vi "Init_UI_Buttons.vi"(0 "VISAResourceName in":refnum<vi>, 1 "Enum Refnum":refnum<vi>, 2 "Bool Refnum 2":refnum<vi>, 3 "Bool Refnum":refnum<vi>, 5 "Str Refnum":refnum<vi>, 7 "DigNum Refnum":refnum<vi>, 9 "DigNum Refnum 2":refnum<vi>, 11 "error in (no error)":errorcluster, 12 "DigNum Refnum 3":refnum<vi>, 13 "Ring Refnum":refnum<vi>) -> (15 "error out":errorcluster)   [LabVIEW 2023, in "TranslationStage Library.lvlib" / "TranslationStage_UI.lvlib" / "TranslationStageUI.lvclass"]
uses:
  TranslationStageUI.lvclass
  TranslationStageUI.lvclass/TranslationStageUI.ctl
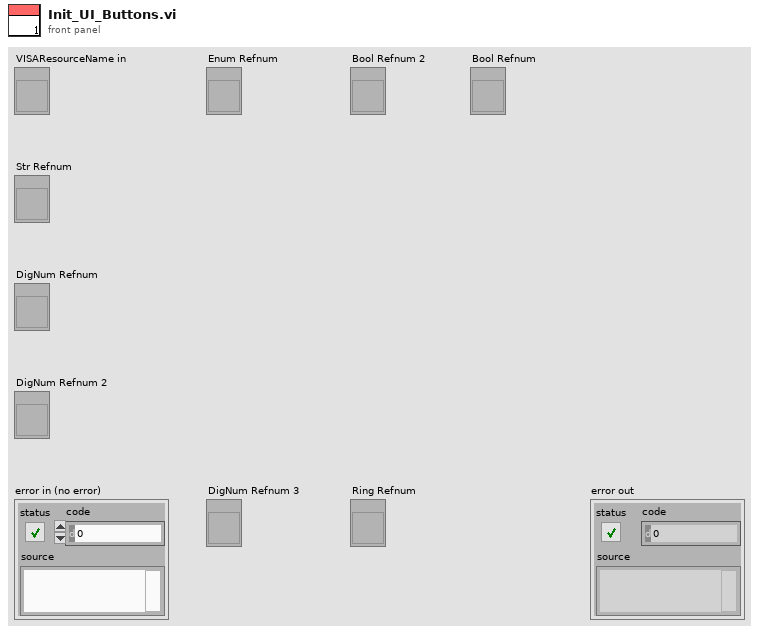
[diagram p1: front panel]
types:
  T1 = enum8{"Enabled", "Disabled", "Disabled and Grayed Out"}
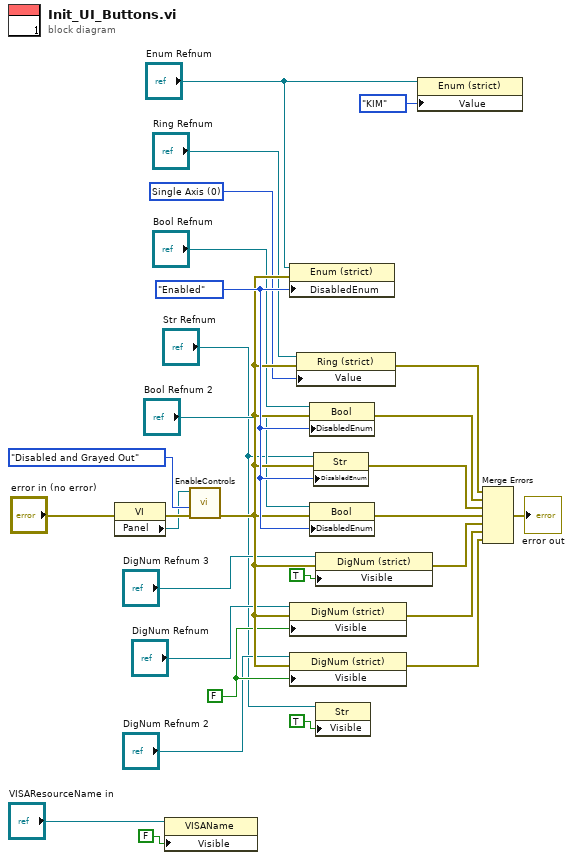
[diagram p0: block diagram]
diagram:
  w16 = 0 items=["Single Axis", "Raster"] ("Scan Mode")
  w15 = FALSE ("Visible")
  w26 = T1."Enabled" ("Disabled")
  n1 = property class="VI"(error in="error in (no error)") -> (error out=w13:errorcluster, "Panel"=w10:refnum<vi>)  [unwired: 1 in, 1 out]
  n2 = property on="Property Node" class="VISAName"(reference="VISAResourceName in", "Visible"=FALSE) -> ()  [unwired: 1 in, 2 out]
  n3 = call "EnableControls.vi"("error in (no error)"=w13, "Disabled"=T1."Disabled and Grayed Out", "Panel in"=w10) -> ("error out"=w25:errorcluster)  [unwired: 8 in]
  n4 = property on="Property Node" class="Enum (strict)"(reference="Enum Refnum", error in=w25, "DisabledEnum"=w26) -> ()  [unwired: 2 out]
  n5 = property on="Property Node" class="DigNum (strict)"(reference="DigNum Refnum", error in=w25, "Visible"=w15) -> (error out=w22:errorcluster)  [unwired: 1 out]
  n6 = property on="Property Node" class="DigNum (strict)"(reference="DigNum Refnum 2", error in=w25, "Visible"=w15) -> (error out=w23:errorcluster)  [unwired: 1 out]
  n7 = property on="Property Node" class="Ring (strict)"(reference="Ring Refnum", error in=w25, "Value"=w16) -> (error out=w17:errorcluster)  [unwired: 1 out]
  n8 = property on="Property Node" class="Bool"(reference="Bool Refnum", error in=w25, "DisabledEnum"=w26) -> (error out=w18:errorcluster)  [unwired: 1 out]
  n9 = property on="Property Node" class="Bool"(reference="Bool Refnum 2", error in=w25, "DisabledEnum"=w26) -> (error out=w20:errorcluster)  [unwired: 1 out]
  n10 = property on="Property Node" class="Str"(reference="Str Refnum", error in=w25, "DisabledEnum"=w26) -> (error out=w19:errorcluster)  [unwired: 1 out]
  n11 = property on="Property Node" class="DigNum (strict)"(reference="DigNum Refnum 3", error in=w25, "Visible"=TRUE) -> (error out=w21:errorcluster)  [unwired: 1 out]
  n12 = property on="Property Node" class="Str"(reference="Str Refnum", "Visible"=TRUE) -> ()  [unwired: 1 in, 2 out]
  n13 = property class="Enum (strict)"(reference="Enum Refnum", "Value"=enum16{"KIM", "Stepper Motors"}."KIM" ("Control")) -> ()  [unwired: 1 in, 2 out]
  n14 = Merge Errors(w17, w18, w19, w20, w21, w22, w23) -> (→"error out":errorcluster)
